vi "Save As Test Executive.vi"(8 "error in (no error)":errorcluster, 10 "Save As Test Executive":T1={"Start Path"=path "", "Pattern (all files)"="", "Pattern Label"="", "Button Label"="", "Default Name"="", "Prompt"="", "Source File"=path "", "Delete Source File?"=FALSE}, 11 "Test Executive Builder Model in":refnum<class "Test Executive Builder Model.lvclass">) -> (0 "error out":errorcluster, 3 "Test Executive Builder Model out":refnum<class "Test Executive Builder Model.lvclass">)   [LabVIEW 2017, in "Test Executive Builder Model.lvclass"]
uses:
  Test Executive Builder Model.lvclass
  <vilib>/gpm_packages/@cs/test-executive/Source/Test Executive/TestExecutive Ref/TestExecutive Ref.lvclass
  Application Dependencies/Save As Test Executive.ctl
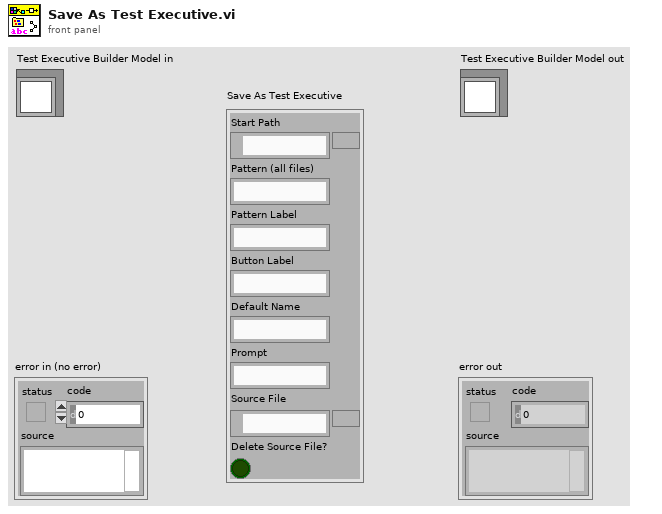
[diagram p1: front panel]
types:
  T1 = typedef "Save As Test Executive.ctl" = cluster{"Start Path":path, "Pattern (all files)":string, "Pattern Label":string, "Button Label":string, "Default Name":string, "Prompt":string, "Source File":path, "Delete Source File?":bool}
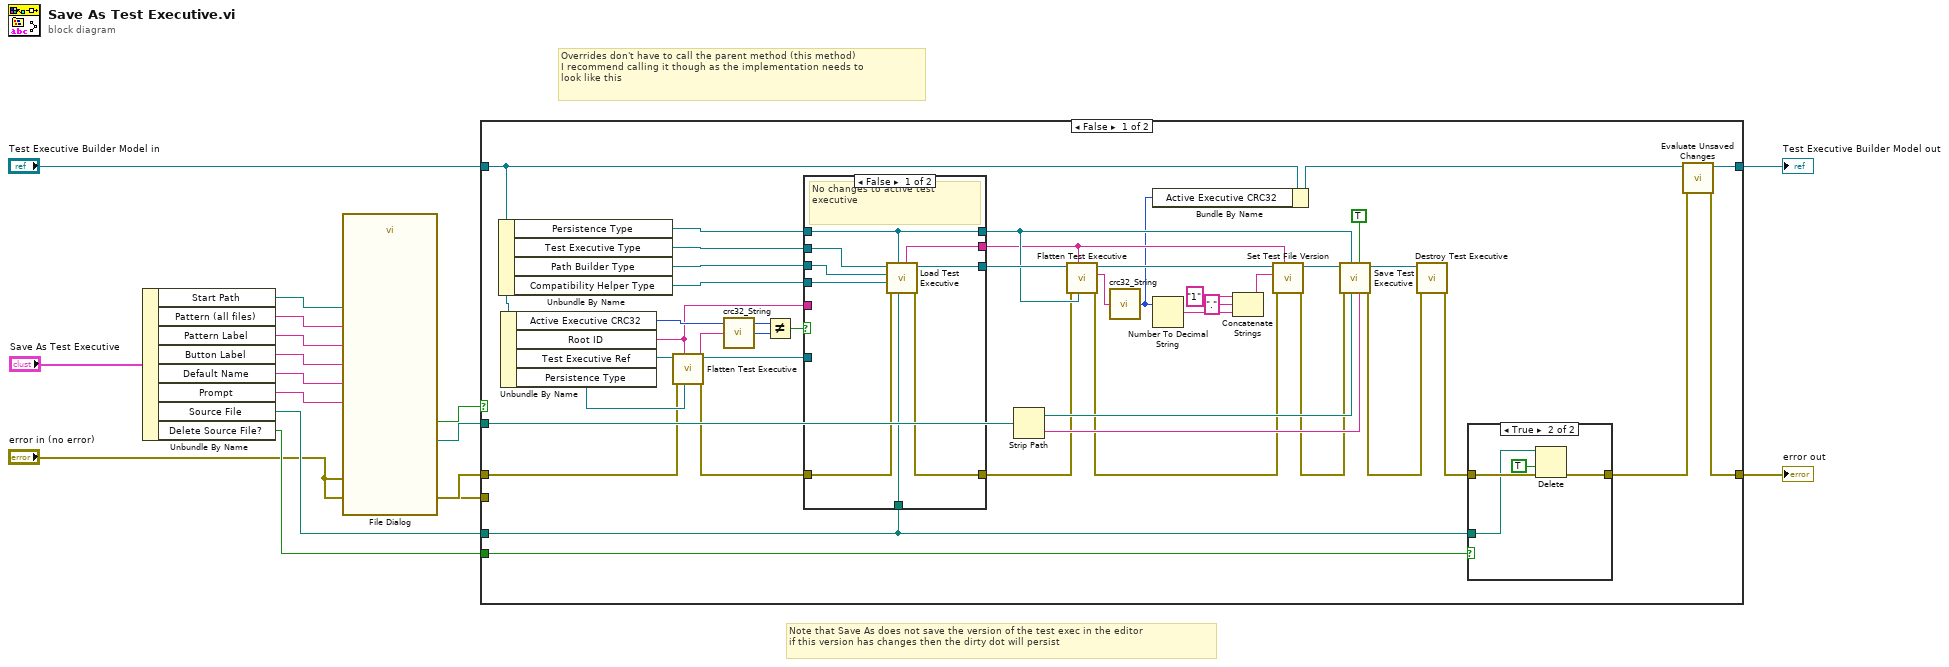
[diagram p0: block diagram]
diagram:
  # "Note that Save As does not save the version of the test exec in the editor\nif this version has changes then the dirty dot will persist"
  # "Overrides don't have to call the parent method (this method)\nI recommend calling it though as the implementation needs to\nlook like this"
  n1 = Unbundle By Name("Save As Test Executive") -> ("Start Path"=w12:path, "Pattern (all files)"=w11:string, "Pattern Label"=w10:string, "Button Label"=w9:string, "Default Name"=w8:string, "Prompt"=w7:string, "Source File"=w2:path, "Delete Source File?"=w3:bool)
  n2 = call "File Dialog"("start path"=w12, "prompt"=w7, "button label"=w9, "default name"=w8, "error in"="error in (no error)", "pattern (all files)"=w11, "pattern label"=w10) -> ("selected path"=w4:path, "cancelled"=w5:bool, "error out"=w6:errorcluster)  [unwired: 5 in, 1 out]
  n3 = case shown="False" w5 {
    tunnel: "Test Executive Builder Model in" -> [w23 w78]
    tunnel: [w19 w78] -> w15
    tunnel: [w18 w77] -> w14
    tunnel: w6 -> [w44 _]
    tunnel: w4 -> [w56 _]
    tunnel: w3 -> [w48 _]
    tunnel: w2 -> [w49 _]
    tunnel: "error in (no error)" -> [_ w77]
    frame False {
      n4 = Unbundle By Name(w23) -> ("Persistence Type"=w39:refnum<class "IPersist.lvclass">, "Test Executive Type"=w55:refnum<class "ITest Executive.lvclass">, "Path Builder Type"=w54:refnum<class "IPath Builder.lvclass">, "Compatibility Helper Type"=w53:refnum<class "ICompatibility Helper.lvclass">)
      n5 = Unbundle By Name(w23) -> ("Active Executive CRC32"=w41:u32, "Root ID"=w37:string, "Test Executive Ref"=w46:refnum<data-value>, "Persistence Type"=w45:refnum<class "IPersist.lvclass">)
      n6 = call <vilib>:"Flatten Test Executive.vi"("Persistence in"=w45, "Root ID"=w37, "error in (no error)"=w44, "Test Executive Ref"=w46) -> ("error out"=w43:errorcluster, "Flattened Test Executive"=w47:string, "Test Executive Ref out"=w38:refnum<data-value>)  [unwired: 5 in]
      n7 = call "crc32_String.vi"("String in"=w47) -> ("CRC32"=w42:u32)  [unwired: 1 in]
      n8 = Not Equal?(x=w41, y=w42) -> (x != y?=w40:bool)
      n9 = case shown="False" w40 {
        tunnel: w39 -> [w60 w70]
        tunnel: w55 -> [w67 _]
        tunnel: w54 -> [w66 _]
        tunnel: w53 -> [w65 _]
        tunnel: [w64 w69] -> w24
        tunnel: [w63 w71] -> w29
        tunnel: w49 -> [w62 _]
        tunnel: w43 -> [w61 w69]
        tunnel: [w60 w70] -> w27
        tunnel: w38 -> [_ w71]
        tunnel: [w59 w68] -> w26
        tunnel: w37 -> [_ w68]
        frame False {
          # "No changes to active test executive"
          n10 = call <vilib>:"Load Test Executive.vi"("Folder"=w62, "Persistence in"=w60, "error in (no error)"=w61, "Compatibility Helper"=w65, "Path Builder"=w66, "Test Executive"=w67) -> ("error out"=w64:errorcluster, "Test Executive Ref out"=w63:refnum<data-value>, "Root ID"=w59:string)  [unwired: 3 in]
        }
        frame True {
          # "Active test exec has been changed, use exec in editor"
        }
      }
      n11 = Strip Path(path=w56) -> (stripped path=w58:path, name=w57:string)
      n12 = call <vilib>:"Flatten Test Executive.vi"("Persistence in"=w27, "Root ID"=w26, "error in (no error)"=w24, "Test Executive Ref"=w29) -> ("error out"=w25:errorcluster, "Flattened Test Executive"=w34:string, "Test Executive Ref out"=w30:refnum<data-value>)  [unwired: 5 in]
      n13 = call "crc32_String.vi"("String in"=w34) -> ("CRC32"=w22:u32)  [unwired: 1 in]
      n14 = Bundle By Name(cluster=w23, "Active Executive CRC32"=w22) -> (w20:refnum<class "Test Executive Builder Model.lvclass">)
      n15 = Number To Decimal String(number=w22) -> (decimal integer string=w32:string)  [unwired: 1 in]
      n16 = Concatenate Strings("1" ("Test File Version"), "." ("string"), w32) -> (w28:string)
      n17 = call <vilib>:"Set Test File Version.vi"("Unique ID"=w26, "error in (no error)"=w25, "Test File Version"=w28, "Test Executive Ref"=w30) -> ("error out"=w35:errorcluster, "Test Executive Ref out"=w36:refnum<data-value>)  [unwired: 6 in]
      n18 = call <vilib>:"Save Test Executive.vi"("File Name"=w57, "New GUIDs"=TRUE, "Folder"=w58, "Persistence in"=w27, "error in (no error)"=w35, "Test Executive Ref"=w36) -> ("error out"=w51:errorcluster, "Test Executive Ref out"=w52:refnum<data-value>)  [unwired: 4 in]
      n19 = call <vilib>:"Destroy Test Executive.vi"("error in (no error)"=w51, "Test Executive Ref"=w52) -> ("error out"=w50:errorcluster)  [unwired: 9 in]
      n20 = case shown="True" w48 {
        tunnel: w50 -> [w72 w76]
        tunnel: [w72 w75] -> w17
        tunnel: w49 -> [_ w74]
        frame False {
        }
        frame True {
          n21 = Delete(path (use dialog)=w74, confirm (F)=TRUE, error in=w76) -> (error out=w75:errorcluster)  [unwired: 2 in, 2 out]
        }
      }
      n22 = call-dynamic "Evaluate Unsaved Changes.vi"("error in (no error)"=w17, "Test Executive Builder Model in"=w20) -> ("error out"=w18:errorcluster, "Test Executive Builder Model out"=w19:refnum<class "Test Executive Builder Model.lvclass">)  [unwired: 8 in]
    }
    frame True {
    }
  }
  "error out" <- w14
  "Test Executive Builder Model out" <- w15
